vi "Calculate Possible Solutions.vi"(10 "Must Contain":T1, 11 "Character Position Possible Letters":T2) -> (2 "Possible Amount":i32, 3 "Possibles":string[](array[string]))   [LabVIEW 2025, in "WordleSolver.lvlib"]
uses:
  WordleSolver.lvlib
  Controls/Character Position Possible Letters.ctl
  Controls/Must Contain.ctl
panel:
  out "Execution Time":dbl
  out "Array":string[][](array[string])
  # "abcdefghijklmnopqrstuvwxyz"
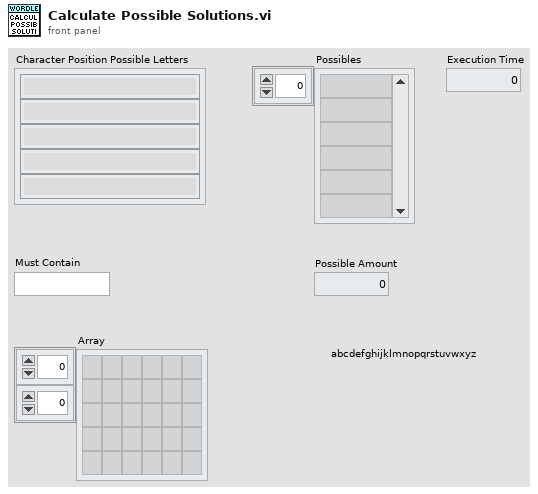
[diagram p1: front panel]
types:
  T1 = typedef "Must Contain.ctl" = string
  T2 = typedef "Character Position Possible Letters.ctl" = string[]
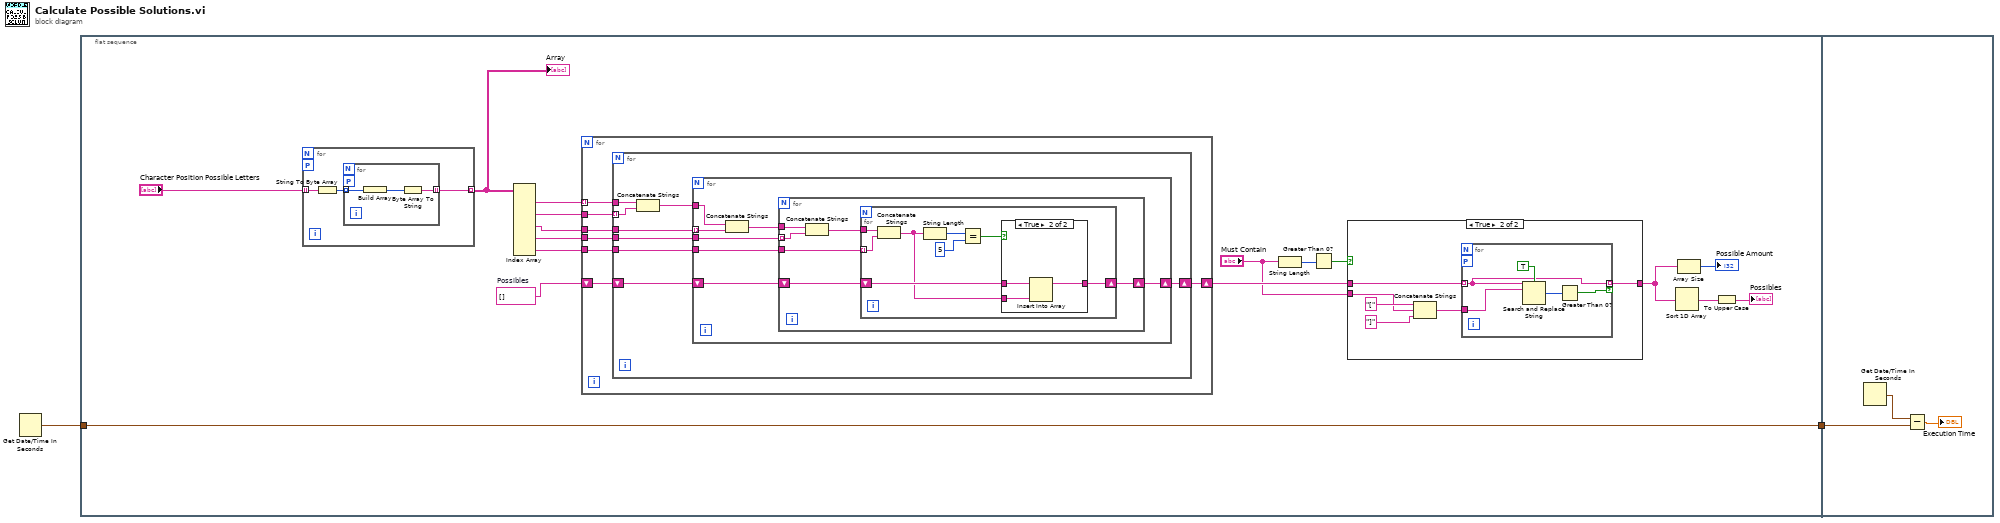
[diagram p0: block diagram]
diagram:
  n1 = Get Date/Time In Seconds() -> (seconds since 1Jan1904=w2:timestamp)
  n2 = flat-sequence {
    tunnel: w2 -> [w4]
    tunnel: [w4] -> w1
    tunnel: w1 -> [w79]
    frame #0 {
      w13 = string[] []  # Possibles
      n3 = for {
        tunnel: "Character Position Possible Letters" -> [w74] mode=indexing
        tunnel: [w72] -> w19 mode=indexing
        workers-P: _ -> [_]
        n4 = String To Byte Array(string=w74) -> (unsigned byte array=w73:u8[])
        n5 = for {
          tunnel: w73 -> [w77] mode=indexing
          tunnel: [w75] -> w72 mode=indexing
          workers-P: _ -> [_]
          n6 = Build Array(w77) -> (w76:u8[])
          n7 = Byte Array To String(unsigned byte array=w76) -> (string=w75:string)
        }
      }
      "Array" <- w19
      n8 = Index Array(array=w19) -> (element #1=w18:string[], element #2=w17:string[], element #3=w16:string[], element #4=w15:string[], element #5=w14:string[])  [unwired: 10 in]
      n9 = for {
        tunnel: w18 -> [w38] mode=indexing
        tunnel: w17 -> [w37]
        tunnel: w16 -> [w36]
        tunnel: w15 -> [w35]
        tunnel: w14 -> [w34]
        shift-right: [w33] -> w10
        shift-left: w13 -> [w32]
        n10 = for {
          tunnel: w38 -> [w46]
          tunnel: w37 -> [w45] mode=indexing
          tunnel: w36 -> [w44]
          tunnel: w35 -> [w43]
          tunnel: w34 -> [w42]
          shift-right: [w41] -> w33
          shift-left: w32 -> [w40]
          n11 = Concatenate Strings(w46, w45) -> (w39:string)
          n12 = for {
            tunnel: w39 -> [w53]
            tunnel: w44 -> [w52] mode=indexing
            tunnel: w43 -> [w51]
            tunnel: w42 -> [w49]
            shift-right: [w48] -> w41
            shift-left: w40 -> [w47]
            n13 = Concatenate Strings(w53, w52) -> (w50:string)
            n14 = for {
              tunnel: w51 -> [w58] mode=indexing
              tunnel: w50 -> [w59]
              tunnel: w49 -> [w56]
              shift-right: [w55] -> w48
              shift-left: w47 -> [w54]
              n15 = Concatenate Strings(w59, w58) -> (w57:string)
              n16 = for {
                tunnel: w57 -> [w67]
                tunnel: w56 -> [w66] mode=indexing
                shift-right: [w65] -> w55
                shift-left: w54 -> [w64]
                n17 = Concatenate Strings(w67, w66) -> (w60:string)
                n18 = String Length(string=w60) -> (length=w62:i32)
                n19 = Equal?(x=w62, y=5) -> (x = y?=w61:bool)
                n20 = case shown="True" w61 {
                  tunnel: [w68 w71] -> w65
                  tunnel: w64 -> [w68 w70]
                  tunnel: w60 -> [_ w69]
                  frame False {
                  }
                  frame True {
                    n21 = Insert Into Array(array=w70, new element=w69) -> (w71:string[])  [unwired: 1 in]
                  }
                }
              }
            }
          }
        }
      }
      n22 = String Length(string="Must Contain") -> (length=w9:i32)
      n23 = Greater Than 0?(x=w9) -> (x > 0?=w8:bool)
      n24 = case shown="True" w8 {
        tunnel: w10 -> [w20 w26]
        tunnel: "Must Contain" -> [_ w22]
        tunnel: [w20 w21] -> w6
        frame False {
        }
        frame True {
          n25 = Concatenate Strings("[" ("string"), w22, "]" ("string")) -> (w23:string)
          n26 = for {
            tunnel: w26 -> [w28] mode=indexing
            tunnel: w23 -> [w31]
            tunnel: [w28] -> w21 mode=indexing if=w27
            workers-P: _ -> [_]
            n27 = Search and Replace String(case sensitive?=TRUE ("ignore case? (F)"), input string=w28, search string=w31) -> (number of replacements=w29:i32)  [unwired: 5 in, 3 out]
            n28 = Greater Than 0?(x=w29) -> (x > 0?=w27:bool)
          }
        }
      }
      n29 = Sort 1D Array(array=w6) -> (sorted array=w11:string[])
      n30 = Array Size(array=w6) -> (size(s)=→"Possible Amount":i32)
      n31 = To Upper Case(1:w11) -> (0:→"Possibles":string[])
    }
    frame #1 {
      n32 = Get Date/Time In Seconds() -> (seconds since 1Jan1904=w80:timestamp)
      n33 = Subtract(x=w80, y=w79) -> (x-y=→"Execution Time":dbl)
    }
  }
